vi "列表框-插入项名.vi"(8 "插入位置（T首，F尾）(F)":bool, 9 "项名":string, 10 "限定行数(500)":u32=500, 11 "LstBox引用句柄":refnum<vi>) -> (3 "引用输出":refnum<vi>)   [LabVIEW 2017]
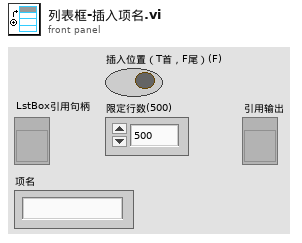
[diagram p1: front panel]
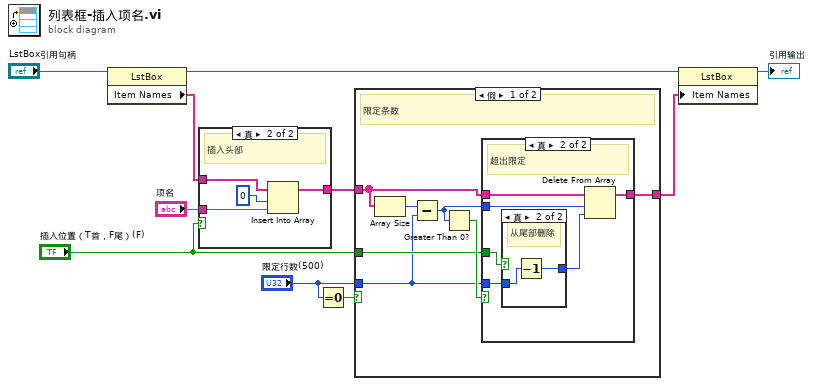
[diagram p0: block diagram]
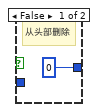
[diagram p3: hidden frame]
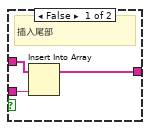
[diagram p5: hidden frame]
diagram:
  n1 = property class="LstBox"(reference="LstBox引用句柄") -> (reference out=w7:refnum<vi>, "Item Names"=w9:string[])  [unwired: 1 in, 1 out]
  n2 = case shown="真" "插入位置（T首，F尾）(F)" {
    tunnel: w9 -> [w13 w17]
    tunnel: "项名" -> [w12 w16]
    tunnel: [w11 w15] -> w5
    frame False {
      # "插入尾部"
      n3 = Insert Into Array(array=w13, new element=w12) -> (w11:string[])  [unwired: 1 in]
    }
    frame True {
      # "插入头部"
      n4 = Insert Into Array(array=w17, index=0 ("索引"), new element=w16) -> (w15:string[])
    }
  }
  n5 = Equal To 0?(x="限定行数(500)") -> (x = 0?=w4:bool)
  n6 = case shown="假" w4 {
    tunnel: w5 -> [w19 w35]
    tunnel: "限定行数(500)" -> [w20 _]
    tunnel: "插入位置（T首，F尾）(F)" -> [w22 _]
    tunnel: [w18 w35] -> w1
    frame False {
      # "限定条数"
      n7 = Array Size(array=w19) -> (size(s)=w23:i32)
      n8 = Subtract(x=w23, y=w20) -> (x-y=w21:u32)
      n9 = Greater Than 0?(x=w21) -> (x > 0?=w24:bool)
      n10 = case shown="真" w24 {
        tunnel: w22 -> [_ w31]
        tunnel: w21 -> [_ w29]
        tunnel: w20 -> [_ w28]
        tunnel: w19 -> [w25 w27]
        tunnel: [w25 w26] -> w18
        frame False {
          # "未超出"
        }
        frame True {
          # "超出限定"
          n11 = case shown="真" w31 {
            tunnel: [0 ("索引") w33] -> w30
            tunnel: w28 -> [_ w34]
            frame False {
              # "从头部删除"
            }
            frame True {
              # "从尾部删除"
              n12 = Decrement(x=w34) -> (x-1=w33:u32)
            }
          }
          n13 = Delete From Array(array=w27, length=w29, index=w30) -> (array with subset deleted=w26:string[])  [unwired: 1 out]
        }
      }
    }
    frame True {
      # "未限定条数"
    }
  }
  n14 = property class="LstBox"(reference=w7, "Item Names"=w1) -> (reference out=→"引用输出":refnum<vi>)  [unwired: 1 in, 1 out]
